vi "CHD_DRIVE_Get_Distances.vi"() -> (1 "RightDistance_M":dbl, 3 "LeftDistance_M":dbl, 4 "MotorDistances_M":dbl[](array[numeric]) format="%17.2f")   [LabVIEW 2019]
uses:
  CHD_DRIVE_GLOBALS.vi
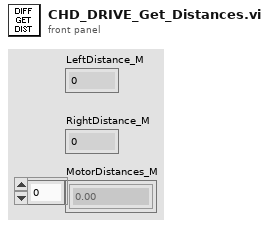
[diagram p1: front panel]
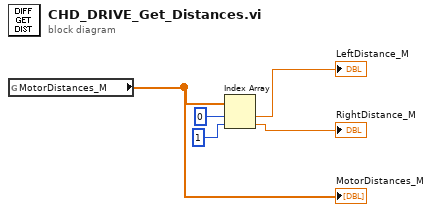
[diagram p0: block diagram]
diagram:
  n1 = global read "CHD_DRIVE_GLOBALS.vi" "MotorDistances_M"() -> (w3:dbl[])
  "MotorDistances_M" <- w3
  n2 = Index Array(array=w3, index #1=0 ("index"), index #2=1 ("index")) -> (element #1=→"LeftDistance_M":dbl, element #2=→"RightDistance_M":dbl)
